vi "SubVI_Downsample_EEG.vi"(8 "error in (no error)":errorcluster, 10 "Resampling rate":dbl, 11 "Filtered EEG in":T2) -> (0 "error out":errorcluster, 3 "Downsampled EEG out":T1)   [LabVIEW 2020]
uses:
  <extravilib>/ChannelInstances/Stream-a[.,.](dbl)/)Channel.ctl
  <extravilib>/ChannelInstances/Stream-a[.](dbl)/)Channel.ctl
  <extravilib>/ChannelInstances/Stream-a[.,.](dbl)/EndpointRead.vi
  <extravilib>/ChannelInstances/Stream-a[.](dbl)/Endpoint.vi
  Global 1.vi
  <extravilib>/ChannelInstances/Stream-a[.,.](dbl)/)Channel.vi
  <resource>/ChannelSupport/_ChannelSupport/WaitIfNeeded.vi
  <extravilib>/ChannelInstances/Stream-a[.](dbl)/)Channel.vi
  <extravilib>/ChannelInstances/Stream-a[.,.](dbl).lvlib
  <extravilib>/ChannelInstances/Stream-a[.](dbl).lvlib
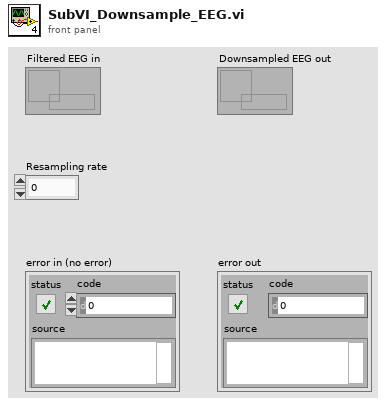
[diagram p1: front panel]
types:
  T1 = typedef "Stream-a[.](dbl).lvlib/)Channel.ctl" = refnum<queue>
  T2 = typedef "Stream-a[.,.](dbl).lvlib/)Channel.ctl" = refnum<queue>
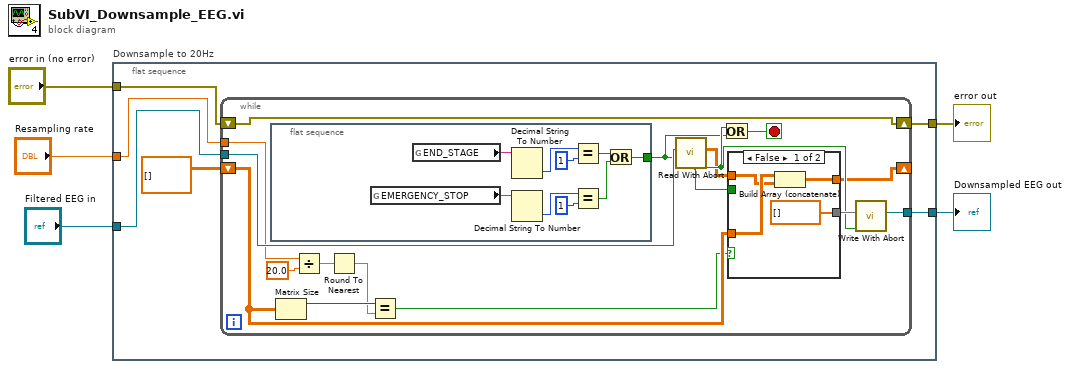
[diagram p0: block diagram]
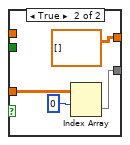
[diagram p2: hidden frame]
diagram:
  n1 = flat-sequence "Downsample to 20Hz" {
    tunnel: [w10] -> w1
    tunnel: [w9] -> w2
    tunnel: "error in (no error)" -> [w8]
    tunnel: "Filtered EEG in" -> [w7]
    tunnel: "Resampling rate" -> [w6]
    frame #0 {
      n2 = while {
        tunnel: w7 -> [w27]
        shift-right: [w12] -> _
        shift-left: dbl[][] [] -> [w26]
        tunnel: w6 -> [w24]
        shift-right: [w18] -> w10
        shift-left: w8 -> [w18]
        tunnel: [w15] -> w9
        stop <- w19 stop-if-true
        n3 = flat-sequence {
          tunnel: [w28] -> w13
          frame #0 {
            n4 = global read "Global 1.vi" "EMERGENCY_STOP"() -> (w31:string)
            n5 = global read "Global 1.vi" "END_STAGE"() -> (w36:string)
            n6 = Decimal String To Number(string=w36) -> (number=w35:i32)  [unwired: 2 in, 1 out]
            n7 = Decimal String To Number(string=w31) -> (number=w33:i32)  [unwired: 2 in, 1 out]
            n8 = Equal?(x=w35, y=1) -> (x = y?=w29:bool)
            n9 = Equal?(x=w33, y=1) -> (x = y?=w30:bool)
            n10 = Or(x=w29, y=w30) -> (x .or. y?=w28:bool)
          }
        }
        n11 = Matrix Size(0:w26) -> (1:w25:i32)  [unwired: 1 out]
        n12 = Divide(x=w24, y=20.0) -> (x/y=w22:dbl)
        n13 = Round To Nearest(number=w22) -> (nearest integer value=w21:dbl)
        n14 = Equal?(x=w25, y=w21) -> (x = y?=w20:bool)
        n15 = call <extravilib>:"Read With Abort.vi"("abort"=w13, "channel"=w27) -> ("element"=w14:dbl[][], "aborted?"=w16:bool)  [unwired: 4 in, 4 out]
        n16 = Or(x=w16, y=w13) -> (x .or. y?=w19:bool)
        n17 = case shown="False" w20 {
          tunnel: w26 -> [w40 w44]
          tunnel: w14 -> [w39 _]
          tunnel: [w38 dbl[][] []] -> w12
          tunnel: w16 -> [_ _]
          tunnel: [dbl[] [] w41] -> w17
          frame False {
            n18 = Build Array (concatenate)(w40, w39) -> (w38:dbl[][])
          }
          frame True {
            n19 = Index Array(array=w44, index (row)=0) -> (element=w41:dbl[])  [unwired: 1 in]
          }
        }
        n20 = call <extravilib>:"Write With Abort.vi"("abort"=w16, "element"=w17) -> ("channel"=w15:T1)  [unwired: 6 in, 3 out]
      }
    }
  }
  "Downsampled EEG out" <- w2
  "error out" <- w1
